vi "Replicate Probability.vi"(11 "Round in":i32) -> (3 "t":dbl)   [LabVIEW 2020, in "Uno.lvclass"]
uses:
  Uno.lvclass
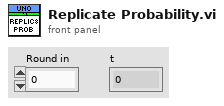
[diagram p1: front panel]
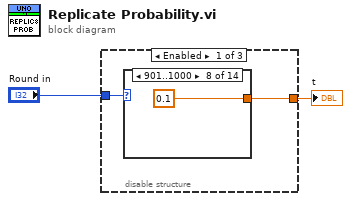
[diagram p0: block diagram]
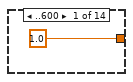
[diagram p2: hidden frame]
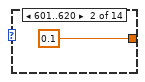
[diagram p3: hidden frame]
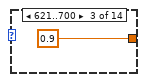
[diagram p4: hidden frame]
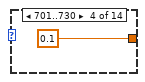
[diagram p5: hidden frame]
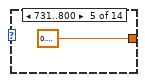
[diagram p6: hidden frame]
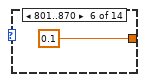
[diagram p7: hidden frame]
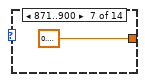
[diagram p8: hidden frame]
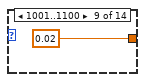
[diagram p9: hidden frame]
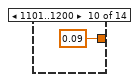
[diagram p10: hidden frame]
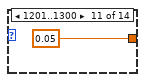
[diagram p11: hidden frame]
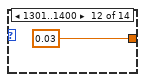
[diagram p12: hidden frame]
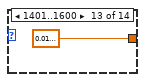
[diagram p13: hidden frame]
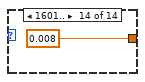
[diagram p14: hidden frame]
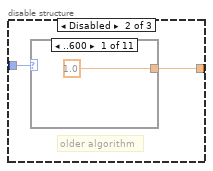
[diagram p15: hidden frame]
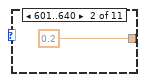
[diagram p16: hidden frame]
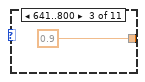
[diagram p17: hidden frame]
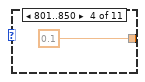
[diagram p18: hidden frame]
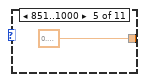
[diagram p19: hidden frame]
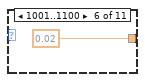
[diagram p20: hidden frame]
diagram:
  n1 = disable-structure shown="Enabled" {
    disable-tunnel: [w4 w20 w33] -> w2
    disable-tunnel: "Round in" -> [w3 w19 w32]
    frame Enabled {
      n2 = case shown="901..1000" w3 {
        tunnel: [1.0 ("t") 0.1 ("t") 0.9 ("t") 0.1 ("t") 0.7999999999999999 ("t") 0.1 ("t") 0.7000000000000001 ("t") 0.1 ("t") 0.02 ("t") 0.09 ("t") 0.05 ("t") 0.03 ("t") 0.010000000000000002 ("t") 0.008 ("t")] -> w4
        frame ..600 {
        }
        frame 601..620 {
        }
        frame 621..700 {
        }
        frame 701..730 {
        }
        frame 731..800 {
        }
        frame 801..870 {
        }
        frame 871..900 {
        }
        frame 901..1000 {
        }
        frame 1001..1100 {
        }
        frame 1101..1200 {
        }
        frame 1201..1300 {
        }
        frame 1301..1400 {
        }
        frame 1401..1600 {
        }
        frame 1601.. {
        }
      }
    }
    frame Disabled {
      # "older algorithm"
      n3 = case shown="..600" w19 {
        tunnel: [1.0 ("t") 0.2 ("t") 0.9 ("t") 0.1 ("t") 0.7000000000000001 ("t") 0.02 ("t") 0.09 ("t") 0.05 ("t") 0.03 ("t") 0.010000000000000002 ("t") 0.008 ("t")] -> w20
        frame ..600 {
        }
        frame 601..640 {
        }
        frame 641..800 {
        }
        frame 801..850 {
        }
        frame 851..1000 {
        }
        frame 1001..1100 {
        }
        frame 1101..1200 {
        }
        frame 1201..1300 {
        }
        frame 1301..1400 {
        }
        frame 1401..1600 {
        }
        frame 1601.. {
        }
      }
    }
    frame Disabled {
      # "experimental"
      n4 = case shown="Default" w32 {
        tunnel: [0.001 ("t") 0.01 ("t")] -> w33
        frame Default {
        }
        frame ..900 {
        }
      }
    }
  }
  "t" <- w2
